vi "Create Channels.vi"(8 "error in (no error)":errorcluster, 10 "Channels":T1[](array[typedef]), 11 "Group Config in":refnum<class "Group Config.lvclass">) -> (0 "error out":errorcluster, 3 "Group Config out":refnum<class "Group Config.lvclass">)   [LabVIEW 2020, in "VectoConfig.lvlib" / "Group Config.lvclass"]
uses:
  Group Config.lvclass
  Channel Init.ctl
  Channel Info.ctl
  Group Config.lvclass/Group Config.ctl
  Channel Config/Channel Config.lvclass
  VectoConfig/VectoConfig.lvlib
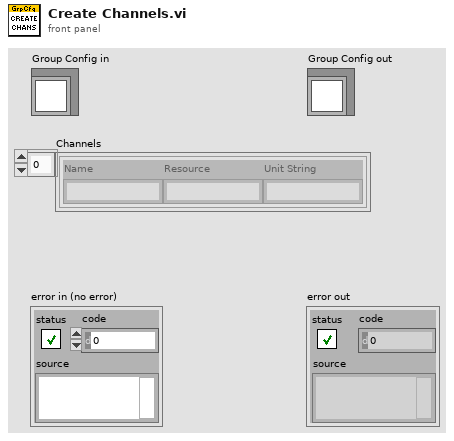
[diagram p1: front panel]
types:
  T1 = typedef "VectoConfig.lvlib/Channel Init.ctl" = cluster{"Name":string, "Resource":string, "Unit String":string}
  T2 = typedef "VectoConfig.lvlib/Channel Info.ctl" = cluster{"Name":string, "Group":string, "Owning Node":string, "Owning Task":string, "Resource":string}
  T3 = typedef "VectoConfig.lvlib/Group Info.ctl" = cluster{"System":string, "Cluster":string, "Node":string, "Task":string, "Name":string}
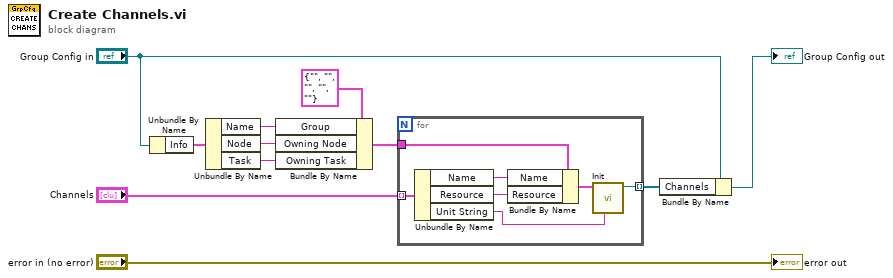
[diagram p0: block diagram]
diagram:
  n1 = Unbundle By Name("Group Config in") -> ("Info"=w9:T3)
  n2 = Unbundle By Name(w9) -> ("Name"=w7:string, "Node"=w6:string, "Task"=w5:string)
  n3 = Bundle By Name(cluster=T2 {"Name"="", "Group"="", "Owning Node"="", "Owning Task"="", "Resource"=""} ("Channel Info"), "Group"=w7, "Owning Node"=w6, "Owning Task"=w5) -> (w3:T2)
  n4 = for {
    tunnel: "Channels" -> [w18] mode=indexing
    tunnel: w3 -> [w17]
    tunnel: [w13] -> w1 mode=indexing
    n5 = Unbundle By Name(w18) -> ("Name"=w16:string, "Resource"=w15:string, "Unit String"=w12:string)
    n6 = Bundle By Name(cluster=w17, "Name"=w16, "Resource"=w15) -> (w14:T2)
    n7 = call "Init.vi"("Unit String (None)"=w12, "Channel Info"=w14) -> ("Channel Config out"=w13:refnum<class "Channel Config.lvclass">)  [unwired: 8 in, 1 out]
  }
  n8 = Bundle By Name(cluster="Group Config in", "Channels"=w1) -> (→"Group Config out":refnum<class "Group Config.lvclass">)
  "error out" <- "error in (no error)"
